vi "svl_Decimation with IC (WDT).vi"(6 "new dt":dbl, 8 "initial decimation state":i32, 9 "init/cont (init:F)":bool, 10 "decimating factor (1)":i32=1 min=1 step=1, 11 "expAveragedArray":waveform(dbl)={"t0"=timestamp(0 s since 1904-01-01), "dt"=0.0, "Y"=[]}) -> (0 "final decimation state":i32, 3 "expAveragedArray":waveform(dbl))   [LabVIEW 2017]
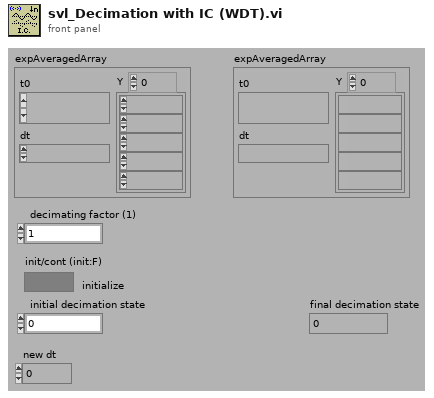
[diagram p1: front panel]
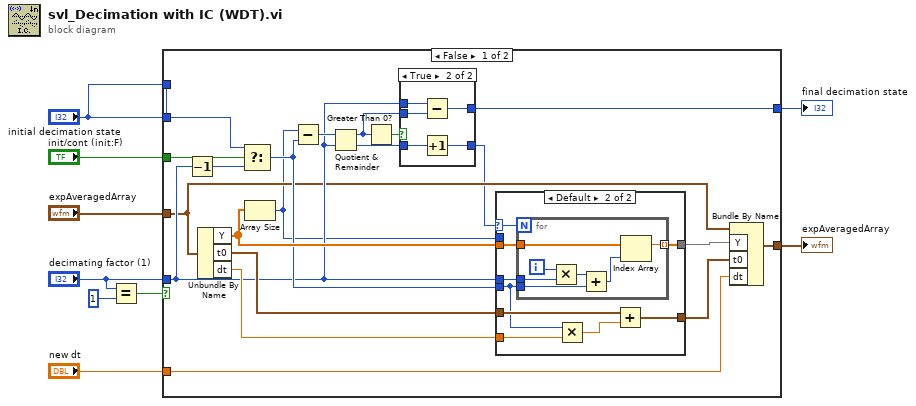
[diagram p0: block diagram]
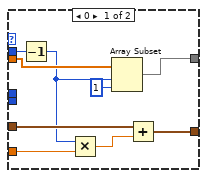
[diagram p2: hidden frame]
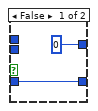
[diagram p3: hidden frame]
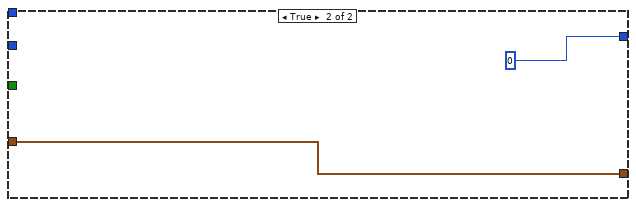
[diagram p4: hidden frame]
diagram:
  n1 = Equal?(x="decimating factor (1)", y=1) -> (x = y?=w6:bool)
  n2 = case shown="False" w6 {
    tunnel: [w20 w63] -> w9
    tunnel: "expAveragedArray" -> [w12 w63]
    tunnel: "initial decimation state" -> [_ _]
    tunnel: "decimating factor (1)" -> [w13 _]
    tunnel: [w25 0] -> w5
    tunnel: "init/cont (init:F)" -> [w24 _]
    tunnel: "initial decimation state" -> [w23 _]
    tunnel: "new dt" -> [w19 _]
    frame False {
      n3 = Decrement(x=w13) -> (x-1=w14:i32)
      n4 = Unbundle By Name(w12) -> ("Y"=w22:dbl[], "t0"=w18:timestamp, "dt"=w17:dbl)
      n5 = Select(t=w23, s=w24, f=w14) -> (s? t:f=w16:i32)
      n6 = Array Size(array=w22) -> (size(s)=w10:i32)
      n7 = Subtract(x=w10, y=w16) -> (x-y=w29:i32)
      n8 = Quotient & Remainder(x=w29, y=w13) -> (x-y*floor(x/y)=w26:i32, floor(x/y)=w27:i32)
      n9 = Greater Than 0?(x=w26) -> (x > 0?=w28:bool)
      n10 = case shown="True" w28 {
        tunnel: w27 -> [w56 w61]
        tunnel: [w56 w60] -> w11
        tunnel: [0 w57] -> w25
        tunnel: w13 -> [_ w59]
        tunnel: w26 -> [_ w58]
        frame False {
        }
        frame True {
          n11 = Subtract(x=w59, y=w58) -> (x-y=w57:i32)
          n12 = Increment(x=w61) -> (x+1=w60:i32)
        }
      }
      n13 = case shown="Default" w11 {
        selector: w11 -> [_ w40]
        tunnel: w22 -> [w33 w47]
        tunnel: [w30 w46] -> w21
        tunnel: w18 -> [w38 w45]
        tunnel: w17 -> [w37 w44]
        tunnel: w16 -> [_ w39]
        tunnel: [w35 w42] -> w15
        tunnel: w13 -> [_ w41]
        tunnel: w10 -> [w34 _]
        frame 0 {
          n14 = Decrement(x=w34) -> (x-1=w32:i32)
          n15 = Multiply(x=w32, y=w37) -> (x*y=w36:dbl)
          n16 = Array Subset(array=w33, index=w32, length=1) -> (w30:dbl[])
          n17 = Add(x=w38, y=w36) -> (x+y=w35:timestamp)
        }
        frame Default {
          n18 = for {
            N: w40 -> [_]
            tunnel: w41 -> [w53]
            tunnel: w47 -> [w54]
            tunnel: w39 -> [w49]
            tunnel: [w48] -> w46 mode=indexing
            i -> [w52]
            n19 = Multiply(x=w52, y=w53) -> (x*y=w51:i32)
            n20 = Add(x=w51, y=w49) -> (x+y=w50:i32)
            n21 = Index Array(array=w54, index=w50) -> (element=w48:dbl)
          }
          n22 = Multiply(x=w39, y=w44) -> (x*y=w43:dbl)
          n23 = Add(x=w45, y=w43) -> (x+y=w42:timestamp)
        }
      }
      n24 = Bundle By Name(cluster=w12, "Y"=w21, "t0"=w15, "dt"=w19) -> (w20:waveform(dbl))
    }
    frame True {
    }
  }
  "expAveragedArray" <- w9
  "final decimation state" <- w5
